vi "Keyence.Main.Scan.Init.vi"(4 "get image":bool, 6 "Retries (-1: Default)":i32=-1, 8 "error in":errorcluster, 9 "ImgPath":path, 10 "Bank":u8, 11 "Data in":T1={"Status"={"State"=enum."Init", "Ref"=refnum, "Bank"=0, "Version"="", "Model"="", "EndTS"=timestamp(0 s since 1904-01-01), "ImgPath"=path "", "Tuned"=FALSE}, "Sets"={"IP"="192.168.2.1", "Timeout_ms"=5000, "Retries"=0, "ReconnectPeriod_s"=0, "ResetPeriod_s"=0, "ReadImg"=FALSE}, "Code"={"text"="", "status"=FALSE, "corners"=[], "level"=0, "class"="", "path"=path ""}}) -> (0 "error out":errorcluster, 2 "started":bool, 3 "Data out":T1={"Status"={"State"=enum."Init", "Ref"=refnum, "Bank"=0, "Version"="", "Model"="", "EndTS"=timestamp(0 s since 1904-01-01), "ImgPath"=path "", "Tuned"=FALSE}, "Sets"={"IP"="192.168.2.1", "Timeout_ms"=5000, "Retries"=0, "ReconnectPeriod_s"=0, "ResetPeriod_s"=0, "ReadImg"=FALSE}, "Code"={"text"="", "status"=FALSE, "corners"=[], "level"=0, "class"="", "path"=path ""}})   [LabVIEW 2016]
uses:
  Keyence.Data.ctl
  Keyence.Data.Status.ctl
  Keyence.Data.Status.State.ctl
  Keyence.Data.Sets.ctl
  LowLevel/Keyence.CodeDetails.ctl
  LowLevel/Keyence.Global.vi
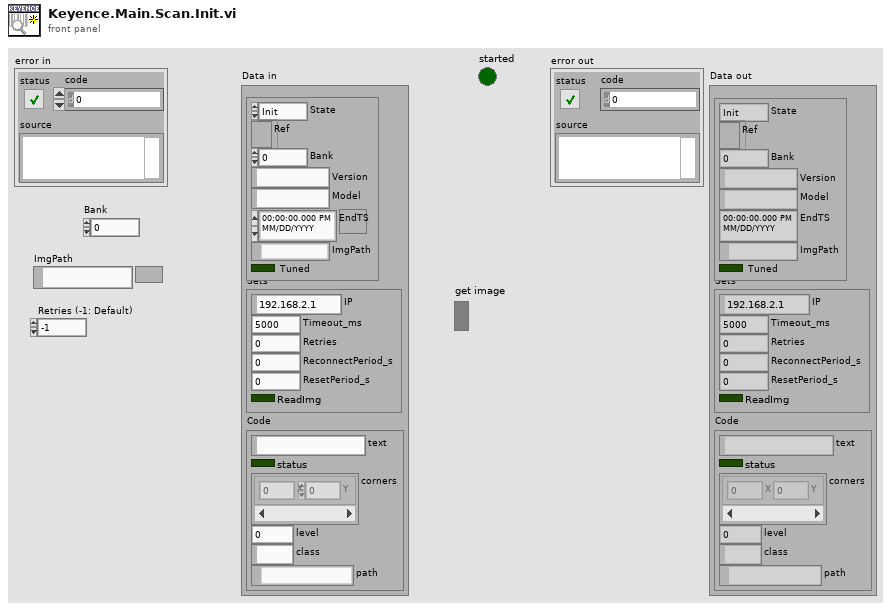
[diagram p1: front panel]
types:
  T1 = typedef "Keyence.Data.ctl" = cluster{"Status":T2, "Sets":T4, "Code":T5}
  T2 = typedef "Keyence.Data.Status.ctl" = cluster{"State":T3, "Ref":refnum<k5>, "Bank":u8, "Version":string, "Model":string, "EndTS":timestamp, "ImgPath":path, "Tuned":bool}
  T3 = typedef "Keyence.Data.Status.State.ctl" = enum16{"First", "Init", "Reset", "Idle", "Scan", "Tune"}
  T4 = typedef "Keyence.Data.Sets.ctl" = cluster{"IP":string, "Timeout_ms":i32, "Retries":i32, "ReconnectPeriod_s":i32, "ResetPeriod_s":i32, "ReadImg":bool}
  T5 = typedef "Keyence.CodeDetails.ctl" = cluster{"text":string, "status":bool, "corners":cluster{"X":i32, "Y":i32}[], "level":u8, "class":string, "path":path}
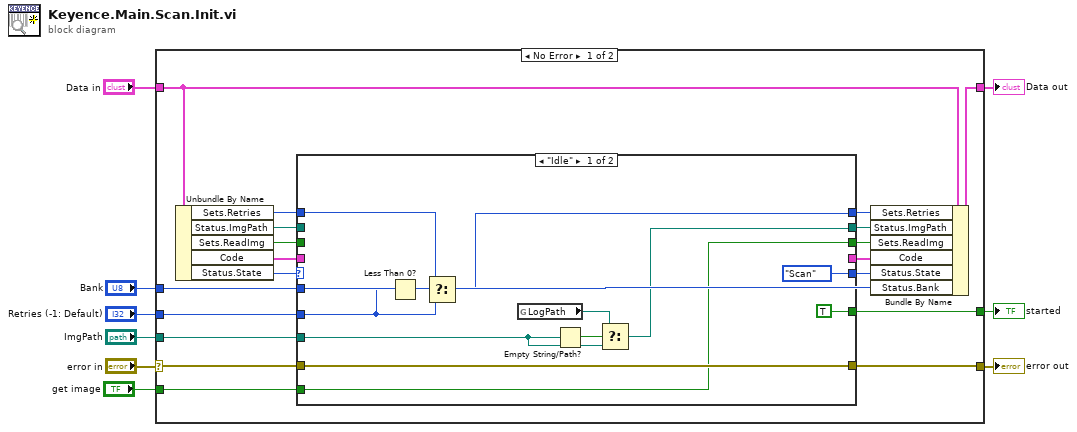
[diagram p0: block diagram]
diagram:
  n1 = case shown="No Error" "error in" {
    selector: "error in" -> [w24 w48]
    tunnel: [w26 w48] -> w6
    tunnel: "Data in" -> [w27 w47]
    tunnel: [w28 w47] -> w7
    tunnel: "Bank" -> [w23 _]
    tunnel: [w19 _] -> w4
    tunnel: "ImgPath" -> [w18 _]
    tunnel: "Retries (-1: Default)" -> [w15 _]
    tunnel: "get image" -> [w10 _]
    frame No Error {
      n2 = Unbundle By Name(w27) -> ("Sets.Retries"=w13:i32, "Status.ImgPath"=w16:path, "Sets.ReadImg"=w12:bool, "Code"=w21:T5, "Status.State"=w25:T3)
      n3 = case shown="\"Idle\"" w25 {
        selector: w25 -> [_ w46]
        tunnel: w24 -> [w39 w44]
        tunnel: [w39 w44] -> w26
        tunnel: w23 -> [_ _]
        tunnel: [Keyence.Data.Status.State."Scan" ("Status.State") w46] -> w22
        tunnel: [_ w45] -> w20
        tunnel: w21 -> [_ w45]
        tunnel: [TRUE _] -> w19
        tunnel: w18 -> [w35 _]
        tunnel: [w34 w43] -> w17
        tunnel: w16 -> [_ w43]
        tunnel: w15 -> [w30 _]
        tunnel: [w31 w42] -> w14
        tunnel: w13 -> [w32 w42]
        tunnel: w12 -> [_ w41]
        tunnel: [w29 w41] -> w11
        tunnel: w10 -> [w29 _]
        frame "Idle" {
          n4 = Less Than 0?(x=w30) -> (x < 0?=w33:bool)
          n5 = Select(t=w32, s=w33, f=w30) -> (s? t:f=w31:i32)
          n6 = global read "Keyence.Global.vi" "LogPath"() -> (w36:path)
          n7 = Empty String/Path?(string/path=w35) -> (empty?=w37:bool)
          n8 = Select(t=w36, s=w37, f=w35) -> (s? t:f=w34:path)
        }
        frame Default {
        }
      }
      n9 = Bundle By Name(cluster=w27, "Sets.Retries"=w14, "Status.ImgPath"=w17, "Sets.ReadImg"=w11, "Code"=w20, "Status.State"=w22, "Status.Bank"=w23) -> (w28:T1)
    }
    frame Error {
    }
  }
  "error out" <- w6
  "Data out" <- w7
  "started" <- w4
